vi "Lab5_PSK2.vi"() -> ()   [LabVIEW 2019]
uses:
  <vilib>/addons/Modulation/Analog/support/mod_Set Error Source.vi
  <vilib>/addons/Modulation/Digital/Support/Common/Validators/mod_AWGN Validate.vi
  <vilib>/addons/Modulation/Digital/Impairments/subVIs/mod_createSeeds.vi
  <vilib>/addons/Modulation/Digital/Support/Common/Validators/mod_Validate Samples Per Symbol.vi
  <vilib>/addons/Modulation/Analog/support/Validators/mod_Validate Complex Waveform.vi
  <vilib>/addons/Modulation/Analog/support/Validators/mod_WFErrorHandler.vi
  <vilib>/addons/Modulation/Digital/General/MT Generate PSK System Parameters(M).vi
  <vilib>/addons/Modulation/Digital/Support/Common/Validators/mod_Generate Filter Coefficients Validate.vi
  <vilib>/addons/Modulation/Digital/General/subVIs/mod_Generate Filter Coefficients.vi
  <vilib>/addons/Modulation/Digital/General/subVIs/mod_Generate Bits PN Sequence.vi
  <vilib>/Analysis/1siggen.llb/Gaussian White Noise (obs 90).vi
  <vilib>/addons/Modulation/Analog/MT Upconvert Baseband (Real).vi
  <vilib>/express/express analysis/Spectral/Block/exnSpectralBlock spectral measurements RMS poly.vi
  <vilib>/express/express analysis/Spectral/Block/exnSpectralBlock spectral measurements RMS WFM.vi
  <vilib>/addons/Modulation/Digital/General/MT Format Eye Diagram (complex).vi
  <vilib>/express/express analysis/Spectral/XNode/ExpressSpectralMeasurementsBlockNode.xnode
  <vilib>/addons/Modulation/niDMT.lvlib
  <vilib>/addons/Modulation/niAMT.lvlib
panel:
  out "Match Found?":bool
  in  "Tab Control":T1(tab)
  out "Spectrum(FFT)":cluster{"f0":dbl, "df":dbl, "magnitude":dbl[]}(graph)
  out "Passband Wfm Spectral Measurements":waveform(dbl)(graph)
  out "Channel Input":cluster{"t0":dbl, "dt":dbl, "Y":dbl[]}(graph)
  out "Channel  Output":cluster{"t0":dbl, "dt":dbl, "Y":dbl[]}(graph)
  in  "stop":bool
  in  "Eb/No(dB)":dbl
  in  "M-PSK":u16(ring) items=["2"=2, "4"=4, "8"=8, "16"=16]
  in  "pulse shaping filter":u16(ring) items=["none", "Raised Cosine", "Root Raised Cos", "Gaussian"]
  in  "Carrier Freq(HZ)":dbl format="%#_2p"
  in  "Symbol Rate(HZ)":dbl format="%#_2p"
  in  "Reset":bool=TRUE
  out "Demodulated String":string
  in  "InputStrig":string
  in  "Add Bit Padding":bool
  in  "Tab Control 2":enum32{"Constellation", "Eye Diagram"}(tab)
  out "PSK Constellation":T2(graph)
  out "Eye Diagram":cluster{"t0":dbl, "dt":dbl, "Y":dbl[]}[](graph)
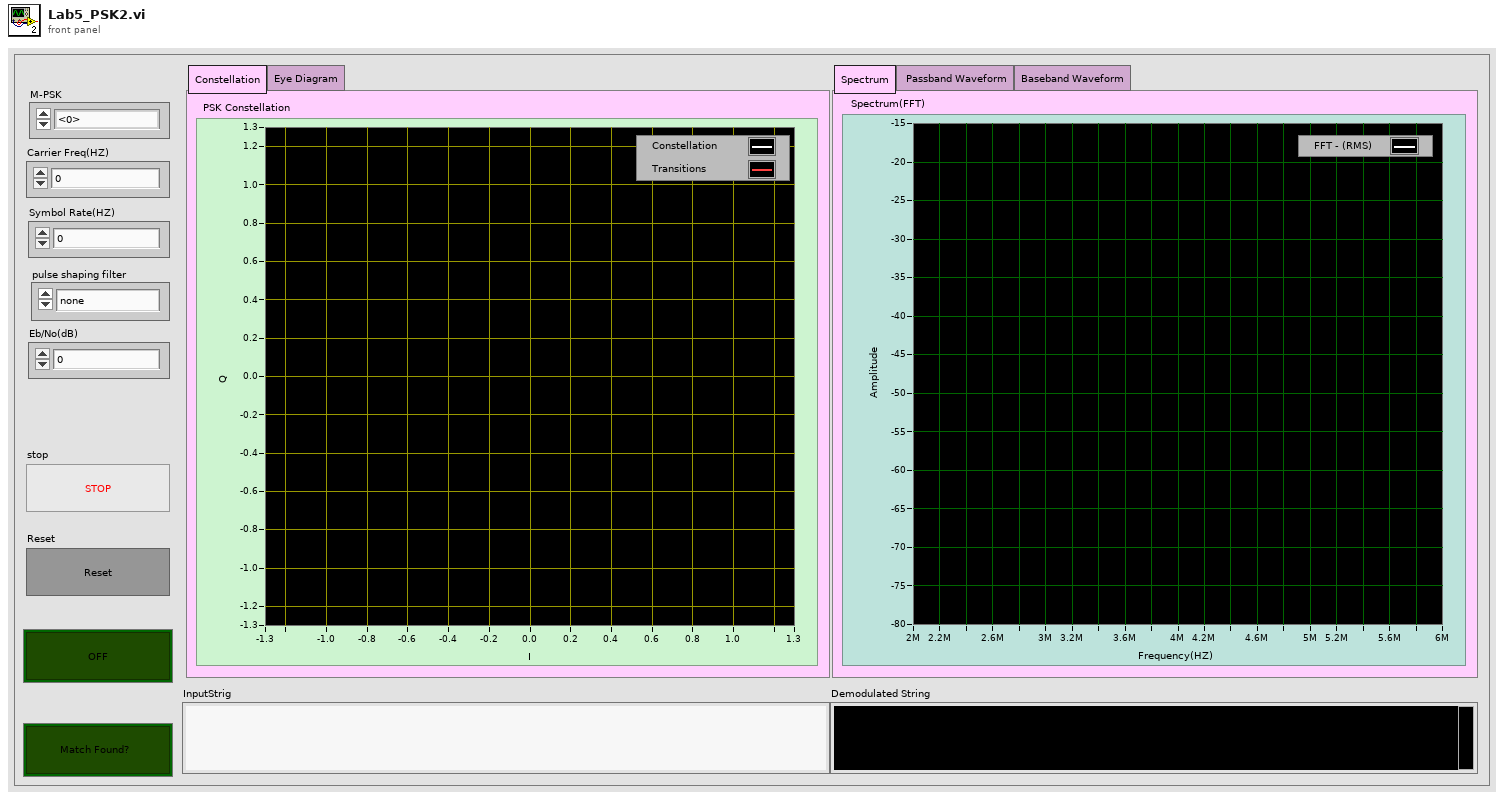
[diagram p1: front panel]
types:
  T1 = enum32{"Spectrum", " Passband Waveform", "Baseband Waveform"}
  T2 = cluster{"Decimated Array":dbl[], "Decimated Array":dbl[]}[]
  T3 = enum16{"FSK", "PSK", "QAM", "MSK", "PAM", "ASK", "CPM"}
  T4 = cluster{"averaging mode":u16, "weighting mode":u16, "number of averages":u32}
  T5 = cluster{"dB On (F)":bool, "unwrap phase (F)":bool, "convert to degree (F)":bool}
  T6 = cluster{"samples per symbol (16)":i32, "symbol map":cdb[], "differential PSK":enum16{"disable", "enable"}, "PSK type":u16}
  T7 = typedef "niAMT.lvlib/Complex Data Waveform.ctl" = cluster{"t0":dbl, "dt":dbl, "Y":cdb[]}
  T8 = cluster{"constellation":dbl[], "oversampled data":dbl[]}[]
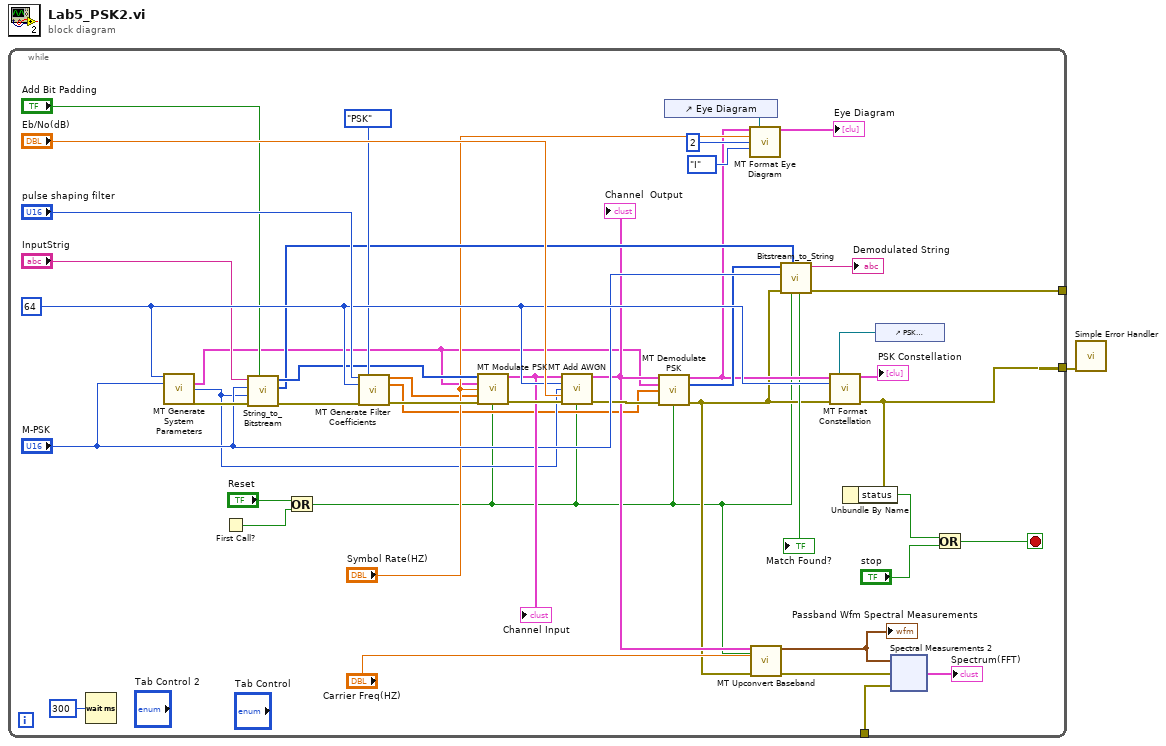
[diagram p0: block diagram]
diagram:
  n1 = while {
    tunnel: [w37] -> w1
    tunnel: [w4] -> _
    tunnel: [w3] -> _
    stop <- w34 stop-if-true
    w40 = 64 ("samples per symbol (16)")
    n2 = Wait (ms)(milliseconds to wait=u32 300) -> ()  [unwired: 1 out]
    n3 = call-poly <vilib>:"MT Generate System Parameters.vi"("samples per symbol (16)"=w40, "M-PSK (4)"="M-PSK") -> ("PSK system parameters"=w11:T6, "bits per symbol"=w16:i32, "error out"=w32:errorcluster)  [unwired: 11 in]
    n4 = First Call?() -> (First Call?: T/F=w30:bool)
    n5 = call "String_to_Bitstream.vi"("Add Bit Padding"="Add Bit Padding", "error in (no error)"=w32, "Guard Bits to Add"=w16, "M-ary (16)"="M-PSK", "InputStrig"="InputStrig") -> ("error out"=w31:errorcluster, "Character Array"=w25:u8[], "Bitstream (with Guard Bits)"=w26:i8[])  [unwired: 1 in, 2 out]
    n6 = Or(x="Reset", y=w30) -> (x .or. y?=w2:bool)
    n7 = call <vilib>:"MT Generate Filter Coefficients.vi"("pulse shaping filter (none)"="pulse shaping filter", "modulation type"=T3."PSK", "pulse shaping samples per symbol (16)"=w40, "error in (no error)"=w31) -> ("pulse shaping filter coefficients"=w9:dbl[], "matched filter coefficients"=w10:dbl[], "error out"=w43:errorcluster)  [unwired: 9 in]
    n8 = call <vilib>:"MT Modulate PSK.vi"("input bit stream"=w26, "PSK system parameters"=w11, "symbol rate (Hz)"="Symbol Rate(HZ)", "pulse shaping filter coefficients"=w9, "error in (no error)"=w43, "reset? (T)"=w2) -> ("output complex waveform"=w38:T7, "error out"=w42:errorcluster)  [unwired: 7 in, 1 out]
    "Channel Input" <- w38
    n9 = call <vilib>:"MT Add AWGN.vi"("input complex waveform"=w38, "samples per symbol (16)"=w40, "bits per symbol (1)"=w16, "Eb/N0 (10 dB)"="Eb/No(dB)", "error in (no error)"=w42, "reset? (T)"=w2) -> ("output complex waveform"=w12:T7, "error out"=w13:errorcluster)  [unwired: 7 in, 1 out]
    "Channel  Output" <- w12
    n10 = call <vilib>:"MT Demodulate PSK.vi"("input complex waveform"=w12, "PSK system parameters"=w11, "matched filter coefficients"=w10, "error in (no error)"=w13, "reset? (T)"=w2) -> ("recovered complex waveform"=w8:T7, "output bit stream"=w15:i8[], "error out"=w6:errorcluster)  [unwired: 6 in, 2 out]
    n11 = control-ref of="Eye Diagram"() -> (w20:refnum<vi>)
    n12 = call-poly <vilib>:"MT Format Eye Diagram.vi"("waveform"=w8, "eye diagram reference"=w20, "symbol rate (Hz)"="Symbol Rate(HZ)", "eye length"=2, "I/Q (I)"=enum16{"I", "Q"}."I") -> ("eye diagram"=→"Eye Diagram":cluster{"t0":dbl, "dt":dbl, "Y":dbl[]}[])  [unwired: 2 in, 8 out]
    n13 = call-poly <vilib>:"MT Upconvert Baseband.vi"("baseband waveform (complex)"=w12, "reset? (F)"=w2, "carrier frequency (Hz)"="Carrier Freq(HZ)", "error in (no error)"=w6) -> ("passband waveform"=w22:waveform(dbl), "error out"=w5:errorcluster)  [unwired: 10 in]
    "Passband Wfm Spectral Measurements" <- w22
    n14 = call "Bitstream_to_String.vi"("Reset"=w2, "Character Array"=w25, "error in (no error)"=w6, "M-ary (16)"="M-PSK", "Bit Array"=w15) -> ("error out"=w3:errorcluster, "Demodulated String"=→"Demodulated String":string, "Match Found?"=→"Match Found?":bool)  [unwired: 1 in, 3 out]
    n15 = control-ref of="PSK Constellation"() -> (w46:refnum<vi>)
    n16 = call <vilib>:"MT Format Constellation.vi"("waveform"=w8, "constellation reference"=w46, "samples per symbol"=w40, "error in (no error)"=w6) -> ("constellation graph"=→"PSK Constellation":T8, "error out"=w37:errorcluster)  [unwired: 1 in, 9 out]
    n17 = Unbundle By Name(w37) -> ("status"=w36:bool)
    n18 = xnode ("Spectral Measurements 2")("Signals"=w22, "error in (no error)"=w5) -> ("FFT - (RMS)"=→"Spectrum(FFT)":cluster{"f0":dbl, "df":dbl, "magnitude":dbl[]}, "error out"=w4:errorcluster)  [unwired: 1 out]
    n19 = Or(x=w36, y="stop") -> (x .or. y?=w34:bool)
  }
  n20 = call <vilib>:"Simple Error Handler.vi"("error in (no error)"=w1) -> ()  [unwired: 4 in, 5 out]
